vi "Filters.vi"(1 "Direction":u16(ring) items=["X-dir", "Y-dir"], 2 "filter type":T2, 3 "Order":dbl=2.0, 7 "Input data":T1, 12 "Sampling Freq":dbl=1000.0, 13 "High Cutoff Freq":dbl=300.0, 14 "Low Cutoff Freq":dbl=50.0) -> (8 "Filterd Data Matrix":T1)   [LabVIEW 2018]
uses:
  <vilib>/Analysis/3filter.llb/Filter Passband Type.ctl
  <vilib>/Analysis/Matrix/Datatypes/RealMatrix.ctl
  <vilib>/Analysis/3filter.llb/Butterworth Filter (DBL).vi
  <vilib>/Analysis/NI_AALBase.lvlib
  <vilib>/Analysis/Matrix/NI_Matrix.lvlib
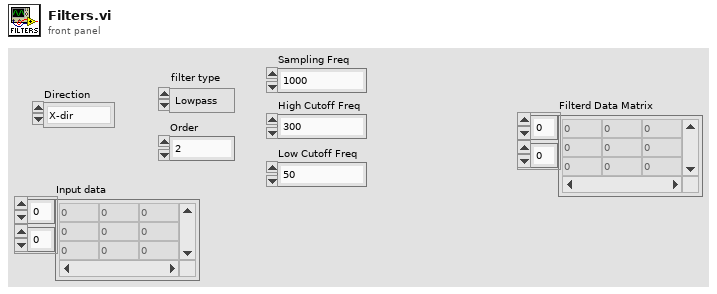
[diagram p1: front panel]
types:
  T1 = typedef "NI_Matrix.lvlib/RealMatrix.ctl" = dbl[][]
  T2 = typedef "NI_AALBase.lvlib/Filter Passband Type.ctl" = enum32{"Lowpass", "Highpass", "Bandpass", "Bandstop"}
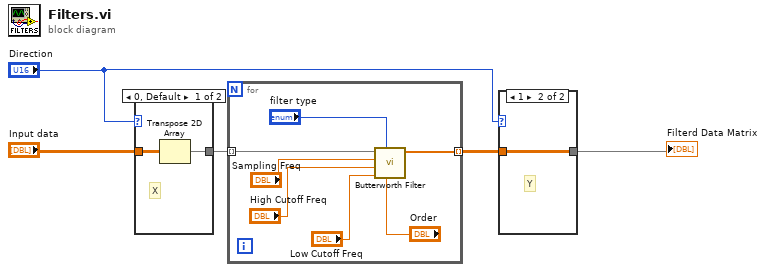
[diagram p0: block diagram]
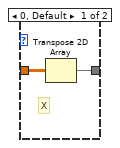
[diagram p2: hidden frame]
diagram:
  n1 = case shown="0, Default" "Direction" {
    tunnel: "Input data" -> [w6 w8]
    tunnel: [w7 w8] -> w5
    frame 0, Default {
      # "X"
      n2 = Transpose 2D Array(2D array=w6) -> (transposed array=w7:T1)
    }
    frame 1 {
      # "Y"
    }
  }
  n3 = for {
    tunnel: w5 -> [w15] mode=indexing
    tunnel: [w10] -> w4 mode=indexing
    n4 = call-poly <vilib>:"Butterworth Filter.vi"("order"="Order", "filter type"="filter type", "low cutoff freq: fl"="Low Cutoff Freq", "high cutoff freq: fh"="High Cutoff Freq", "sampling freq: fs"="Sampling Freq", "X"=w15) -> ("Filtered X"=w10:dbl[])  [unwired: 2 in, 1 out]
  }
  n5 = case shown="1" "Direction" {
    tunnel: w4 -> [w16 w18]
    tunnel: [w17 w18] -> w1
    frame 0, Default {
      # "X"
      n6 = Transpose 2D Array(2D array=w16) -> (transposed array=w17:dbl[][])
    }
    frame 1 {
      # "Y"
    }
  }
  "Filterd Data Matrix" <- w1
